vi "Shut Down Device.vi"(8 "error in (no error)":errorcluster, 11 "Photometrics Camera in":refnum<class "Photometrics Camera.lvclass">) -> (0 "error out":errorcluster, 3 "Photometrics Camera out":refnum<class "Photometrics Camera.lvclass">)   [LabVIEW 2023, in "Photometrics Camera.lvlib" / "Photometrics Camera.lvclass"]
uses:
  Photometrics Camera.lvclass
  Photometrics Camera.lvclass/Photometrics Camera.ctl
  Users/Public/Documents/Photometrics/TPM-LabVIEWSamples BETA/TPM LabVIEW adapter/Camera/Camera.lvclass
  Camera/Camera.lvclass
  Users/Public/Documents/Photometrics/TPM-LabVIEWSamples BETA/TPM LabVIEW adapter/PVCAM/PVCAM.lvclass
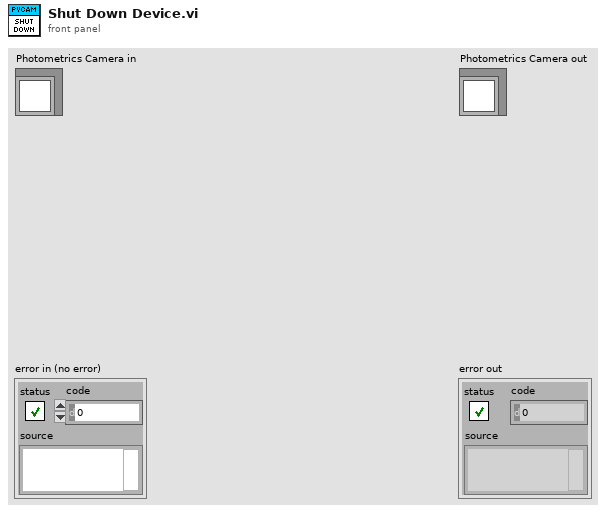
[diagram p1: front panel]
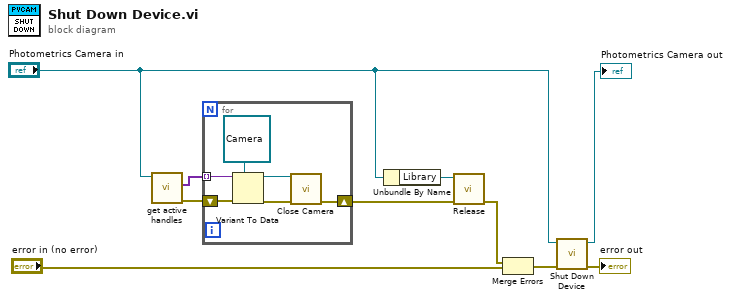
[diagram p0: block diagram]
diagram:
  n1 = call-dynamic "get active handles.vi"("Camera in"="Photometrics Camera in") -> ("error out"=w5:errorcluster, "Handles"=w8:variant[])  [unwired: 6 in, 3 out]
  n2 = for {
    tunnel: w8 -> [w16] mode=indexing
    shift-right: [w13] -> w4
    shift-left: w5 -> [w11]
    n3 = Variant To Data(error in=w11, type=refnum<class "Camera.lvclass"> refnum ("Camera out"), Variant=w16) -> (data=w14:refnum<class "Camera.lvclass">, error out=w12:errorcluster)
    n4 = call "Close Camera.vi"("error in (no error)"=w12, "Camera in"=w14) -> ("error out"=w13:errorcluster)  [unwired: 8 in, 1 out]
  }
  n5 = Unbundle By Name("Photometrics Camera in") -> ("Library"=w6:refnum<class "PVCAM.lvclass">)
  n6 = call "Release.vi"("error in (no error)"=w4, "PVCAM in"=w6) -> ("error out"=w1:errorcluster)  [unwired: 8 in, 1 out]
  n7 = Merge Errors(w1, "error in (no error)") -> (w3:errorcluster)
  n8 = call-parent "Shut Down Device.vi"("error in (no error)"=w3, "Device in"="Photometrics Camera in") -> ("error out"=→"error out":errorcluster, "Device out"=→"Photometrics Camera out":refnum<class "Photometrics Camera.lvclass">)  [unwired: 8 in]
